vi "FrequencySet_HT.vi"(6 "error in":errorcluster, 9 "VCO Frequency":i32=2400) -> (0 "error out":errorcluster)   [LabVIEW 2011]
doc: "This VI sets the frequency of the HT Link 0 PLL instance.\n\nInputs:\n1. Frequency: Selects the frequency that the HT PLL will be set to."
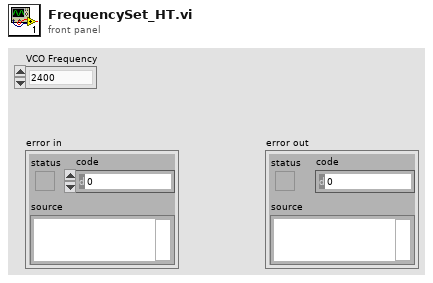
[diagram p1: front panel]
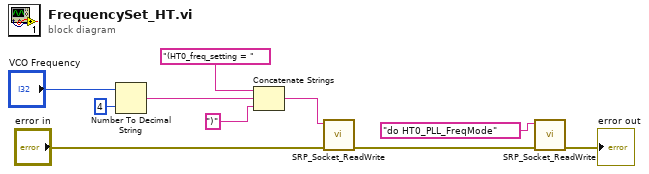
[diagram p0: block diagram]
diagram:
  n1 = Number To Decimal String ("HT Link 0 PLL Frequency")(number="VCO Frequency", width (-)=i16 4) -> (decimal integer string=w6:string)
  n2 = Concatenate Strings("(HT0_freq_setting = ", w6, ")") -> (w2:string)
  n3 = call "SRP_Socket_ReadWrite.vi"("error in (no error)"="error in", "Data In"=w2) -> ("error out"=w4:errorcluster)  [unwired: 7 in, 1 out]
  n4 = call "SRP_Socket_ReadWrite.vi"("error in (no error)"=w4, "Data In"="do HT0_PLL_FreqMode") -> ("error out"=→"error out":errorcluster)  [unwired: 7 in, 1 out]
